vi "Read Bus Monitor Interface.vi"(10 "Datum Name":string, 11 "ListboxBusMonitor":refnum<class "ListboxBusMonitor.lvclass">) -> (2 "Valid Transport":refnum<class "ITransport.lvclass">, 3 "SubscriptionPolicy Type":refnum<class "ISubscriptionPolicy.lvclass">)   [LabVIEW 2020, in "ListboxBusMonitor.lvlib" / "ListboxBusMonitor.lvclass"]
uses:
  <vilib>/gpm_packages/@cs/BusMonitor/ListboxBusMonitor/ListboxBusMonitor/ListboxBusMonitor.lvclass
  <vilib>/gpm_packages/@cs/transport/Source/ITransport/ITransport.lvclass
  <vilib>/gpm_packages/@cs/mva-core/Source/IMediator/ISubscriptionPolicy/ISubscriptionPolicy.lvclass
  <vilib>/gpm_packages/@cs/BusMonitor/ListboxBusMonitor/ListboxBusMonitor/ListboxBusMonitor.lvclass/ListboxBusMonitor.ctl
  <vilib>/gpm_packages/@cs/mva-core/Source/SubscriptionPolicy/BasicSubscription/BasicSubscription.lvclass/BasicSubscription.ctl
  <vilib>/gpm_packages/@cs/BusMonitor/ListboxBusMonitor/ListboxBusMonitorPanel Messages/Update Monitored Datum Msg/Update Monitored Datum Msg.lvclass
  C:/Program Files/National Instruments/LabVIEW 2020/vi.lib/gpm_packages/@cs/transport/Source/Concrete/ActorMessageTransport/Notification Msg/Notification Msg.lvclass
  <vilib>/gpm_packages/@cs/transport/Source/Concrete/ActorMessageTransport/ActorMessageTransport.lvclass/ActorMessageTransport.ctl
  <vilib>/ActorFramework/Message Enqueuer/Equals Not A Refnum.vi
  <vilib>/gpm_packages/@cs/mva-core/Source/SubscriptionPolicy/BasicSubscription/BasicSubscription.lvclass
  C:/Program Files/National Instruments/LabVIEW 2020/vi.lib/gpm_packages/@cs/mva-core/Source/IMediator/ISubscriptionPolicy/ISubscriptionPolicy.lvclass
  <vilib>/gpm_packages/@cs/transport/Source/Concrete/ActorMessageTransport/ActorMessageTransport.lvclass
  C:/Program Files/National Instruments/LabVIEW 2020/vi.lib/gpm_packages/@cs/transport/Source/ITransport/ITransport.lvclass
  <vilib>/Utility/error.llb/Error Cluster From Error Code.vi
  <vilib>/ActorFramework/Message Enqueuer/Message Enqueuer.lvclass
  <vilib>/gpm_packages/@cs/transport/Source/Concrete/ActorMessageTransport/Notification Msg/Notification Msg.lvclass
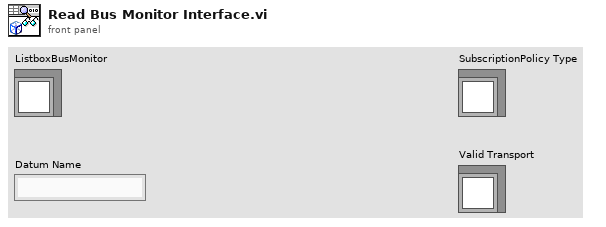
[diagram p1: front panel]
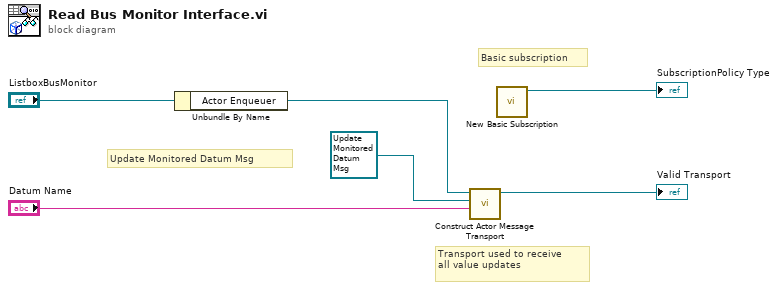
[diagram p0: block diagram]
diagram:
  # "Basic subscription"
  # "Transport used to receive\nall value updates"
  # "Update Monitored Datum Msg"
  n1 = Unbundle By Name("ListboxBusMonitor") -> ("Actor Enqueuer"=w5:refnum<class "Message Enqueuer.lvclass">)
  n2 = call <vilib>:"Construct Actor Message Transport.vi"("Datum Name"="Datum Name", "Notification Msg"=refnum<class "Update Monitored Datum Msg.lvclass"> refnum ("ListboxBusMonitor.lvlib:Update Monitored Datum Msg.lvclass"), "Message Enqueuer in"=w5) -> ("ActorMessageTransport"=→"Valid Transport":refnum<class "ActorMessageTransport.lvclass">)  [unwired: 7 in, 1 out]
  n3 = call <vilib>:"New Basic Subscription.vi"() -> ("BasicSubscription Out"=→"SubscriptionPolicy Type":refnum<class "BasicSubscription.lvclass">)  [unwired: 11 in]
